vi "P4CMD Initialize.vi"(8 "error in (no error)":errorcluster, 11 "provider name":string="Perforce Command Line") -> (0 "error out":errorcluster, 2 "suppCaps":u32)   [LabVIEW 2020, in "NI_SCC_P4CMD.lvlib"]
uses:
  <vilib>/SourceControl/Providers/P4CMD/NI_SCC_P4CMD.lvlib
  <vilib>/SourceControl/support/SCCSup ConfigData Conv.ctl
  <vilib>/SourceControl/Providers/P4CMD/P4CMD Mgr Functions.ctl
  <vilib>/SourceControl/Providers/P4CMD/P4CMD Advanced Options.ctl
  <vilib>/SourceControl/support/SCCSup Message Strings GLBL.vi
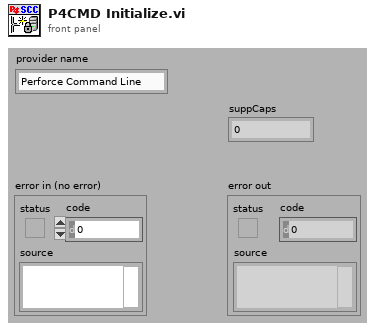
[diagram p1: front panel]
types:
  T1 = typedef "NI_SCC_P4CMD.lvlib/P4CMD Advanced Options.ctl" = cluster{"lock files?":bool, "suppress dialogs?":bool}
  T2 = typedef "NI_SCC_P4CMD.lvlib/P4CMD Mgr Functions.ctl" = enum16{"Init", "Open", "Set Config Opts", "Initialized?", "IsRefValid?", "Get Config Opts", "Get Global Commands", "Close", "Uninit"}
  T3 = typedef "SCCSup ConfigData Conv.ctl" = enum16{"from config data", "to config data"}
  T4 = typedef "NI_SCC_P4CMD.lvlib/P4CMD SCC Config Info.ctl" = cluster{"GBL lock on checkout?":bool, "GBL suppress dlgs?":bool, "port":string, "client":string, "user":string, "password":string}
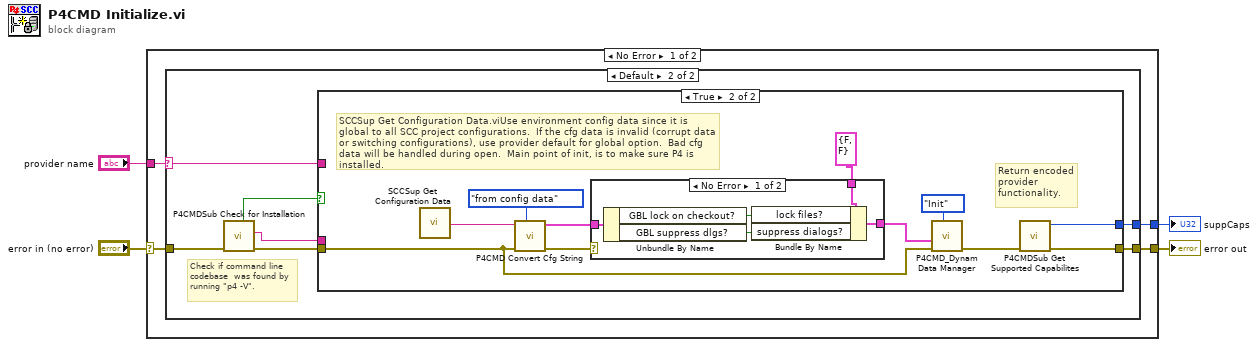
[diagram p0: block diagram]
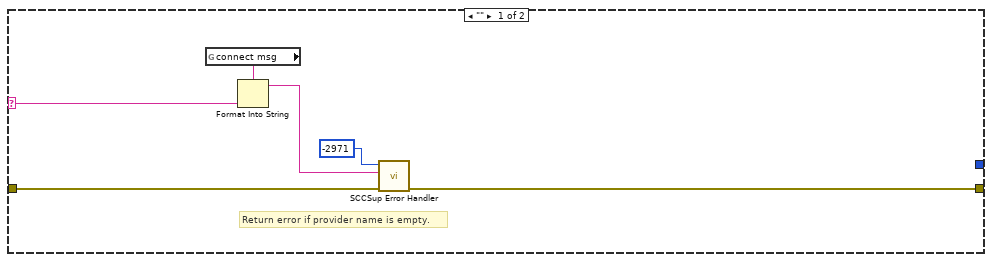
[diagram p2: hidden frame]
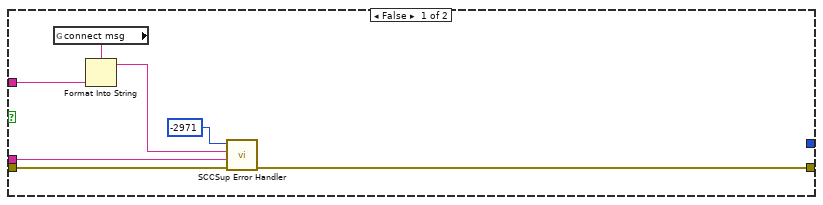
[diagram p3: hidden frame]
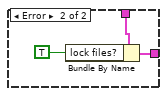
[diagram p4: hidden frame]
diagram:
  n1 = case shown="No Error" "error in (no error)" {
    selector: "error in (no error)" -> [w8 w48]
    tunnel: [w7 w48] -> w2
    tunnel: "provider name" -> [w6 _]
    tunnel: [w5 _] -> w1
    frame No Error {
      n2 = case shown="Default" w6 {
        selector: w6 -> [w9 w16]
        tunnel: w8 -> [w11 w21]
        tunnel: [w10 w17] -> w7
        tunnel: [_ w15] -> w5
        frame "" {
          # "Return error if provider name is empty."
          n3 = global read "SCCSup Message Strings GLBL.vi" "connect msg"() -> (w13:string)
          n4 = Format Into String(format string=w13, w9) -> (resulting string=w12:string)  [unwired: 2 in, 1 out]
          n5 = call <vilib>:"SCCSup Error Handler.vi"("error in (no error)"=w11, "operation message"=w12, "scc error code"=-2971 ("t")) -> ("error out"=w10:errorcluster)  [unwired: 8 in]
        }
        frame Default {
          # "Check if command line codebase  was found by running \"p4 -V\"."
          n6 = call <vilib>:"P4CMDSub Check for Installation.vi"("error in (no error)"=w21) -> ("error out"=w19:errorcluster, "path info"=w18:string, "Perforce installed?"=w20:bool)  [unwired: 8 in]
          n7 = case shown="True" w20 {
            tunnel: w19 -> [w28 w32]
            tunnel: w18 -> [w27 _]
            tunnel: [w25 w31] -> w17
            tunnel: w16 -> [w23 _]
            tunnel: [_ w30] -> w15
            frame False {
              n8 = global read "SCCSup Message Strings GLBL.vi" "connect msg"() -> (w24:string)
              n9 = Format Into String(format string=w24, w23) -> (resulting string=w22:string)  [unwired: 2 in, 1 out]
              n10 = call <vilib>:"SCCSup Error Handler.vi"("error in (no error)"=w28, "additional message"=w27, "operation message"=w22, "scc error code"=-2971 ("t")) -> ("error out"=w25:errorcluster)  [unwired: 7 in]
            }
            frame True {
              # "SCCSup Get Configuration Data.viUse environment config data since it is global to all SCC project configurations.  If the cfg data is invalid (corrupt data or switching configurations), use provider default for global option.  Bad cfg data will be handled during open.  Main point of init, is to make sure P4 is installed."
              # "Return encoded provider functionality."
              n11 = call <vilib>:"SCCSup Get Configuration Data.vi"() -> ("configuration data"=w29:string)  [unwired: 6 in]
              n12 = call <vilib>:"P4CMD Convert Cfg String.vi"("conversion action"=SCCSup_ConfigData_Conv."from config data", "error in (no error)"=w32, "config data in"=w29) -> ("error out"=w37:errorcluster, "configuration details out"=w38:T4)  [unwired: 6 in, 1 out]
              n13 = case shown="No Error" w37 {
                tunnel: w38 -> [w44 _]
                tunnel: [w40 w46] -> w35
                tunnel: T1 {"lock files?"=FALSE, "suppress dialogs?"=FALSE} ("adv cfg options in") -> [w43 w47]
                frame No Error {
                  n14 = Unbundle By Name(w44) -> ("GBL lock on checkout?"=w42:bool, "GBL suppress dlgs?"=w41:bool)
                  n15 = Bundle By Name(cluster=w43, "lock files?"=w42, "suppress dialogs?"=w41) -> (w40:T1)
                }
                frame Error {
                  n16 = Bundle By Name(cluster=w47, "lock files?"=TRUE) -> (w46:T1)
                }
              }
              n17 = call <vilib>:"P4CMD_Dynam Data Manager.vi"("function"=P4CMD_Mgr_Functions."Init", "error in (no error)"=w32, "adv cfg options in"=w35) -> ("error out"=w33:errorcluster)  [unwired: 3 in, 5 out]
              n18 = call <vilib>:"P4CMDSub Get Supported Capabilites.vi"("error in (no error)"=w33) -> ("error out"=w31:errorcluster, "suppCaps"=w30:u32)  [unwired: 9 in]
            }
          }
        }
      }
    }
    frame Error {
    }
  }
  "error out" <- w2
  "suppCaps" <- w1
